vi "Copy Help.vi"(8 "Error In":errorcluster, 11 "Target Project Root In":path) -> (0 "Error Out":errorcluster, 3 "Target Project Root Out":path)   [LabVIEW 2017, in "Scripts.lvlib"]
doc: "Copies the `src\\Help` folder to the target destination. This is necessary because the Save for Previous operation does not automatically copy the `Help` folder and its contents to the target destination. The Help source is NOT included in the project file because it would be a hassle to include all of the files using virtual folders."
uses:
  Scripts.lvlib
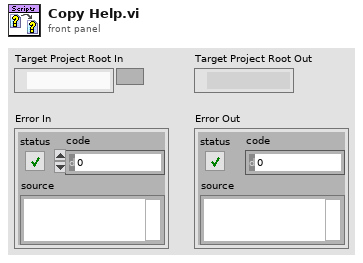
[diagram p1: front panel]
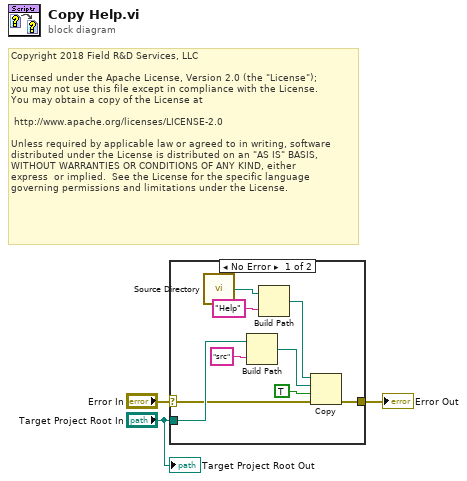
[diagram p0: block diagram]
diagram:
  # "Copyright 2018 Field R&D Services, LLC\n\nLicensed under the Apache License, Version 2.0 (the \"License\");\nyou may not use this file except in compliance with the License.\nYou may obtain a copy of the License at\n\n\thttp://www.apache.org/licenses/LICENSE-2.0\n\nUnless required by applicable law or agreed to in writing, software\ndistributed under the License is distributed on an \"AS IS\" BASIS,\nWITHOUT WARRANTIES OR CONDITIONS OF ANY KIND, either \nexpress  or implied.  See the License for the specific language \ngoverning permissions and limitations under the License."
  n1 = case shown="No Error" "Error In" {
    selector: "Error In" -> [w5 w13]
    tunnel: "Target Project Root In" -> [w12 _]
    tunnel: [w11 w13] -> w2
    frame No Error {
      n2 = call "Source Directory.vi"() -> ("Source Directory"=w6:path)
      n3 = Build Path(base path=w12, name or relative path="src") -> (appended path=w10:path)
      n4 = Build Path(base path=w6, name or relative path="Help") -> (appended path=w8:path)
      n5 = Copy(8:w5, 9:TRUE ("overwrite (F)"), 10:w10, 11:w8) -> (0:w11:errorcluster)  [unwired: 1 in, 2 out]
    }
    frame Error {
    }
  }
  "Error Out" <- w2
  "Target Project Root Out" <- "Target Project Root In"
